vi "3_采集图像并保存.vi"() -> ()   [LabVIEW 2020]
uses:
  <vilib>/vision/driver/NI_Vision_Acquisition_Software.lvlib
panel:
  out "真":bool
  in  "存储照片":bool
  out "Image":T1(plugin-control)
  in  "停止":bool
  out "错误信息显示":errorcluster
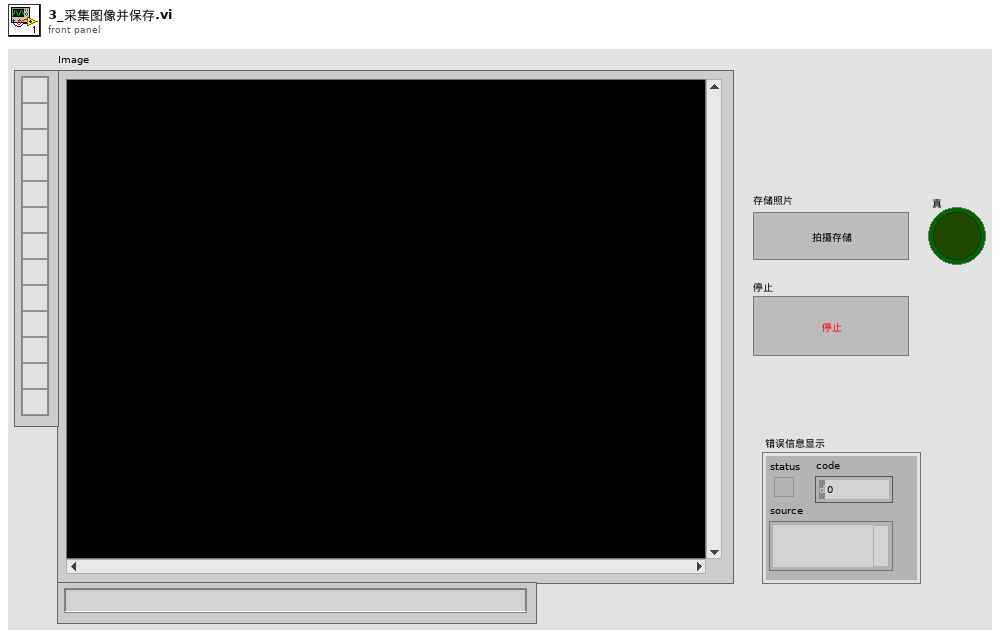
[diagram p1: front panel]
types:
  T1 = typedef "IMAQ Image.ctl" = refnum<image>
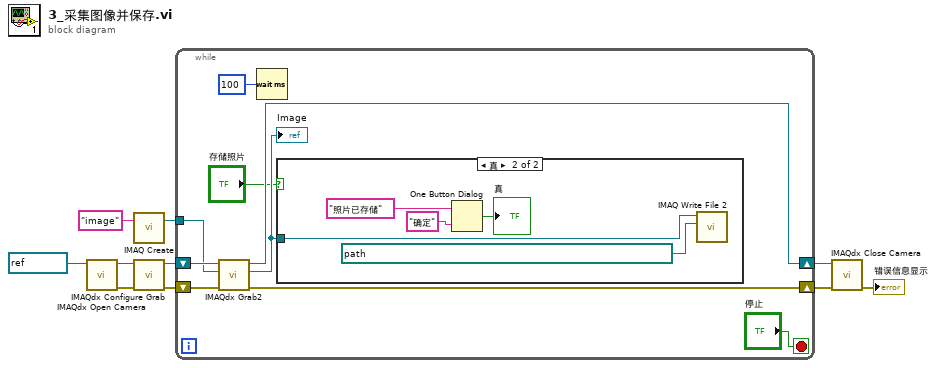
[diagram p0: block diagram]
diagram:
  n1 = call <vilib>:"IMAQdx Open Camera.vi"("Session In"=refnum<k21> "cam0") -> ("error out"=w9:errorcluster, "Session Out"=w10:refnum<k21>)  [unwired: 9 in]
  n2 = call "IMAQ Create"("Image Name"="image") -> ("New Image"=w5:T1)  [unwired: 4 in, 1 out]
  n3 = call <vilib>:"IMAQdx Configure Grab.vi"("error in"=w9, "Session In"=w10) -> ("error out"=w8:errorcluster, "Session Out"=w7:refnum<k21>)  [unwired: 8 in]
  n4 = while {
    shift-right: [w15] -> w2
    shift-left: w8 -> [w19]
    shift-right: [w16] -> w3
    shift-left: w7 -> [w18]
    tunnel: w5 -> [w17]
    stop <- "停止" stop-if-true
    n5 = call <vilib>:"IMAQdx Grab2.vi"("error in"=w19, "Image In"=w17, "Session In"=w18) -> ("error out"=w15:errorcluster, "Image Out"=w13:T1, "Session Out"=w16:refnum<k21>)  [unwired: 5 in, 1 out]
    "Image" <- w13
    n6 = Wait (ms)(milliseconds to wait=u32 100 ("等待时间（毫秒）")) -> ()  [unwired: 1 out]
    n7 = case shown="真" "存储照片" {
      tunnel: w13 -> [_ w23]
      frame False {
      }
      frame True {
        n8 = One Button Dialog(message="照片已存储" ("消息"), button name ("OK")="确定" ("按钮名称（“确定”）")) -> (true=→"真":bool)
        n9 = call-poly "IMAQ Write File 2"("File Path"=path "D:/Labview/LabView_program/1_1_图片路径/image.png", "Image"=w23) -> ()  [unwired: 8 in, 2 out]
      }
    }
  }
  n10 = call <vilib>:"IMAQdx Close Camera.vi"("error in"=w2, "Session In"=w3) -> ("error out"=→"错误信息显示":errorcluster)  [unwired: 9 in]
